vi "Read NumberOfRobots.vi"(8 "error in (no error)":errorcluster, 11 "PreparePenaltyAllyPlay in":refnum<class "PreparePenaltyAllyPlay.lvclass">) -> (0 "error out":errorcluster, 2 "NumberOfRobots":dbl=5.0, 3 "PreparePenaltyAllyPlay out":refnum<class "PreparePenaltyAllyPlay.lvclass">)   [LabVIEW 2023, in "PreparePenaltyAllyPlay.lvclass"]
uses:
  PreparePenaltyAllyPlay.lvclass
  PreparePenaltyAllyPlay.lvclass/PreparePenaltyAllyPlay.ctl
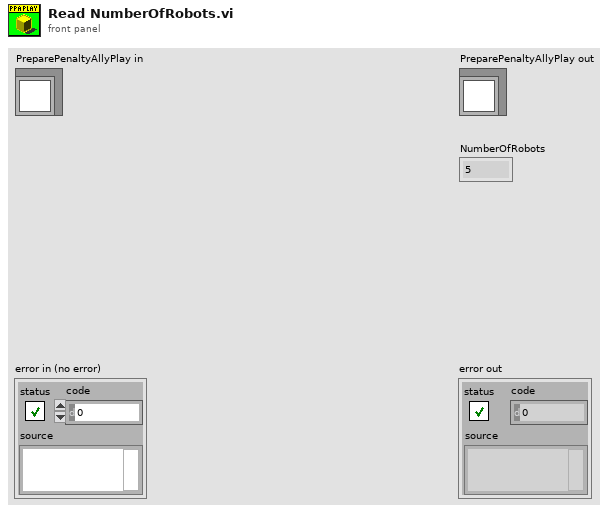
[diagram p1: front panel]
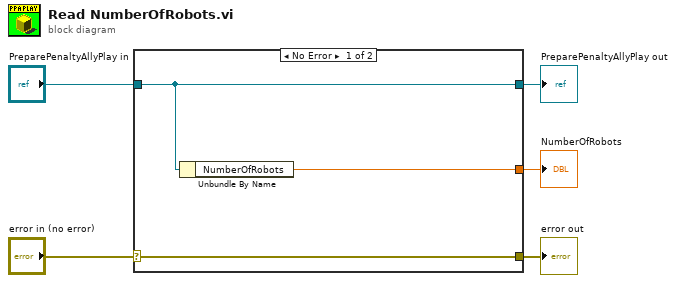
[diagram p0: block diagram]
diagram:
  n1 = case shown="No Error" "error in (no error)" {
    selector: "error in (no error)" -> [w8 w9]
    tunnel: [w8 w9] -> w4
    tunnel: [w7 w10] -> w2
    tunnel: "PreparePenaltyAllyPlay in" -> [w7 w10]
    tunnel: [w6 _] -> w1
    frame No Error {
      n2 = Unbundle By Name(w7) -> ("NumberOfRobots"=w6:dbl)
    }
    frame Error {
    }
  }
  "error out" <- w4
  "PreparePenaltyAllyPlay out" <- w2
  "NumberOfRobots" <- w1
